vi "Main Engine Data Log Folder Check.vi"(8 "error in":errorcluster) -> (0 "error out":errorcluster)   [LabVIEW 2021]
doc: "All Rights Reserved © 2023 SyncSols"
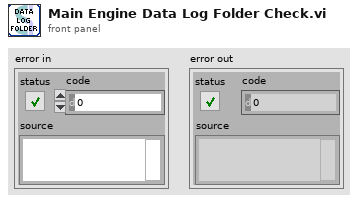
[diagram p1: front panel]
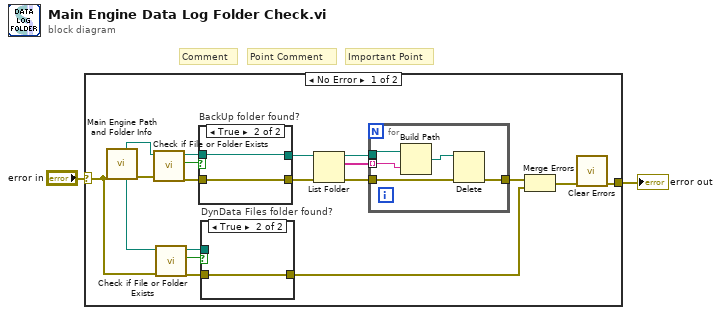
[diagram p0: block diagram]
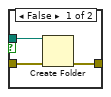
[diagram p2: hidden frame]
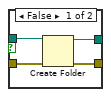
[diagram p3: hidden frame]
diagram:
  # "Important Point"
  # "Point Comment"
  # "Comment"
  n1 = case shown="No Error" "error in" {
    selector: "error in" -> [w5 w37]
    tunnel: [w12 w37] -> w2
    frame No Error {
      n2 = call "Main Engine Path and Folder Info.vi"("error in"=w5) -> ("error out"=w7:errorcluster, "DynData File"=w6:path, "Data Logging"=w18:path)  [unwired: 5 in, 3 out]
      n3 = call <vilib>:"Check if File or Folder Exists.vi"("error in (no error)"=w7, "path"=w18) -> ("error out"=w19:errorcluster, "file or folder exists?"=w21:bool, "dup path"=w20:path)  [unwired: 7 in]
      n4 = call <vilib>:"Check if File or Folder Exists.vi"("error in (no error)"=w5, "path"=w6) -> ("error out"=w10:errorcluster, "file or folder exists?"=w8:bool, "dup path"=w9:path)  [unwired: 7 in]
      n5 = case "BackUp folder found?" shown="True" w21 {
        tunnel: w20 -> [w34 w36]
        tunnel: w19 -> [w33 w35]
        tunnel: [w32 w36] -> w11
        tunnel: [w31 w35] -> w17
        frame False {
          n6 = Create Folder(path (use dialog)=w34, error in=w33) -> (created path=w32:path, error out=w31:errorcluster)  [unwired: 1 in, 1 out]
        }
        frame True {
        }
      }
      n7 = case "DynData Files folder found?" shown="True" w8 {
        tunnel: w9 -> [w24 _]
        tunnel: w10 -> [w23 w25]
        tunnel: [w22 w25] -> w3
        frame False {
          n8 = Create Folder(path (use dialog)=w24, error in=w23) -> (error out=w22:errorcluster)  [unwired: 1 in, 2 out]
        }
        frame True {
        }
      }
      n9 = List Folder(path=w11, error in=w17) -> (path out=w16:path, filenames=w15:string[], error out=w14:errorcluster)  [unwired: 2 in, 1 out]
      n10 = for {
        tunnel: w16 -> [w30]
        tunnel: w15 -> [w29] mode=indexing
        tunnel: w14 -> [w28]
        tunnel: [w27] -> w13
        n11 = Build Path(base path=w30, name or relative path=w29) -> (appended path=w26:path)
        n12 = Delete(path (use dialog)=w26, error in=w28) -> (error out=w27:errorcluster)  [unwired: 3 in, 2 out]
      }
      n13 = Merge Errors(w13, w3) -> (w4:errorcluster)
      n14 = call <vilib>:"Clear Errors.vi"("error in (no error)"=w4) -> ("error out"=w12:errorcluster)  [unwired: 5 in, 1 out]
    }
    frame Error {
    }
  }
  "error out" <- w2
